vi "trigger.vi"() -> (14 "triggered":bool)   [LabVIEW 2014]
uses:
  triggerGlobalVars.vi
  Sequencer/sequencerGlobVars.vi
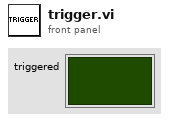
[diagram p1: front panel]
types:
  T1 = typedef "selectTrigger.ctl" = enum8{"Ext0", "Ext1", "Ext2", "Ext3", "Ext4", "Ext5", "Ext6", "Ext7", "Int0", "Int1", "Int2", "Int3", "Int4", "Int5", "Int6", "Int7"}
  T2 = typedef "triggerTypes.ctl" = enum16{"noTrigger", "singleHitDelay", "singleHit", "software", "sweep"}
  T3 = typedef "triggerEdge.ctl" = enum8{"either", "false-true", "true-false"}
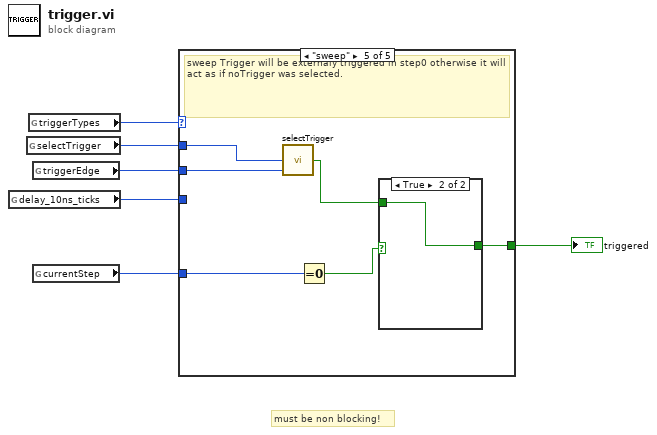
[diagram p0: block diagram]
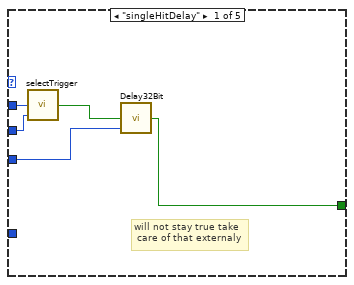
[diagram p2: hidden frame]
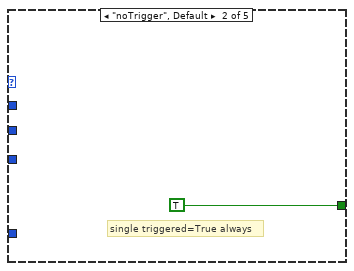
[diagram p3: hidden frame]
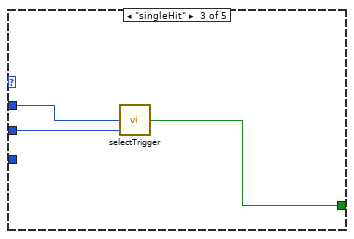
[diagram p4: hidden frame]
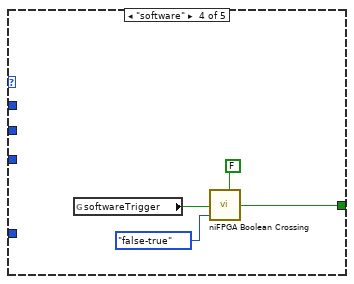
[diagram p5: hidden frame]
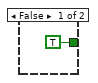
[diagram p6: hidden frame]
diagram:
  # "must be non blocking!"
  n1 = global read "triggerGlobalVars.vi" "delay_10ns_ticks"() -> (w3:u32)
  n2 = global read "triggerGlobalVars.vi" "selectTrigger"() -> (w4:T1)
  n3 = global read "triggerGlobalVars.vi" "triggerTypes"() -> (w5:T2)
  n4 = global read "triggerGlobalVars.vi" "triggerEdge"() -> (w2:T3)
  n5 = global read "sequencerGlobVars.vi" "currentStep"() -> (w1:i32)
  n6 = case shown="\"sweep\"" w5 {
    tunnel: w4 -> [w11 _ w15 _ w25]
    tunnel: w3 -> [w9 _ _ _ _]
    tunnel: [w8 TRUE w13 w19 w20] -> w6
    tunnel: w2 -> [w7 _ w14 _ w24]
    tunnel: w1 -> [_ _ _ _ w23]
    frame "singleHitDelay" {
      # "will not stay true take\n care of that externaly"
      n7 = call "selectTrigger.vi"("triggerEdge"=w7, "MCSSelectTrigger"=w11) -> ("fired"=w10:bool)  [unwired: 3 in]
      n8 = call "Delay32Bit.vi"("delay(ticks)"=w9, "In"=w10) -> ("Out"=w8:bool)  [unwired: 3 in]
    }
    frame "noTrigger", Default {
      # "single triggered=True always"
    }
    frame "singleHit" {
      n9 = call "selectTrigger.vi"("triggerEdge"=w14, "MCSSelectTrigger"=w15) -> ("fired"=w13:bool)  [unwired: 3 in]
    }
    frame "software" {
      n10 = global read "triggerGlobalVars.vi" "softwareTrigger"() -> (w18:bool)
      n11 = call <vilib>:"niFPGA Boolean Crossing.vi"("input"=w18, "direction"=enum8{"either", "false-true", "true-false"}."false-true", "initialize"=FALSE) -> ("crossing"=w19:bool)  [unwired: 6 in]
    }
    frame "sweep" {
      # "sweep Trigger will be externaly triggered in step0 otherwise it will act as if noTrigger was selected."
      n12 = call "selectTrigger.vi"("triggerEdge"=w24, "MCSSelectTrigger"=w25) -> ("fired"=w21:bool)  [unwired: 3 in]
      n13 = Equal To 0?(x=w23) -> (x = 0?=w22:bool)
      n14 = case shown="True" w22 {
        tunnel: w21 -> [_ w27]
        tunnel: [TRUE ("fired") w27] -> w20
        frame False {
        }
        frame True {
        }
      }
    }
  }
  "triggered" <- w6
